vi "生成报表.vi"() -> ()   [LabVIEW 2013]
panel:
  in  "error in (no error) 2":errorcluster={"status"=TRUE, "code"=51111, "source"="路径不存在"}
  in  "error in (no error)":errorcluster={"status"=TRUE, "code"=51111, "source"="路径不存在"}
  out "String":string
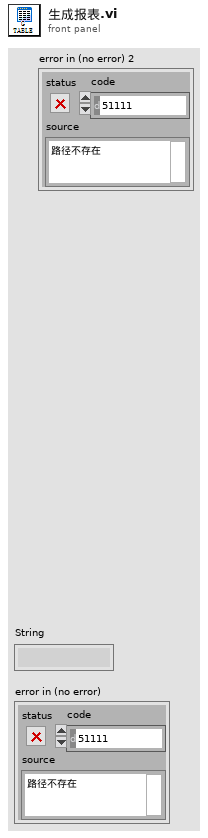
[diagram p1: front panel]
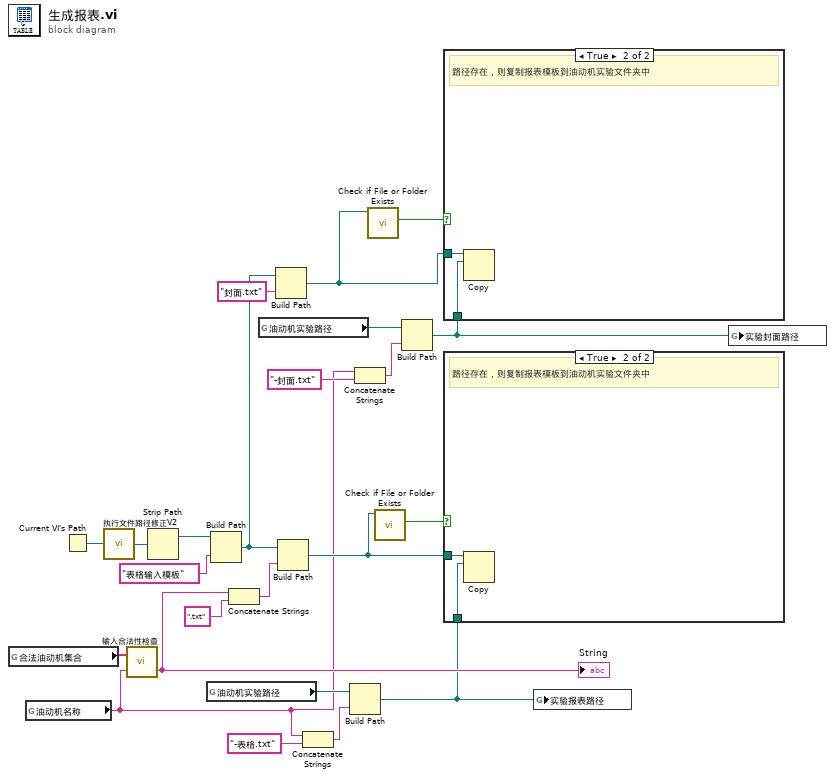
[diagram p0: block diagram]
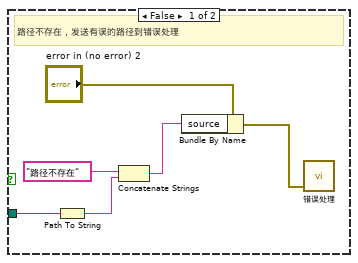
[diagram p2: hidden frame]
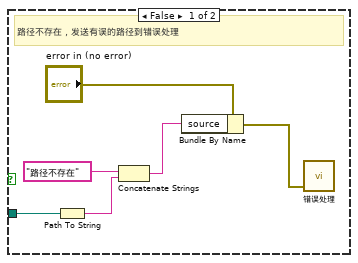
[diagram p3: hidden frame]
diagram:
  n1 = global read "合法油动机集合.vi" "合法油动机集合"() -> (w23:string[])
  n2 = global read "油动机名称.vi" "油动机名称"() -> (w2:string)
  n3 = Current VI's Path() -> (path=w11:path)
  n4 = call "执行文件路径修正V2.vi"("Path in"=w11) -> ("Path out"=w10:path)
  n5 = call "输入合法性检查.vi"("被检查名称"=w2, "合法名称集合"=w23) -> ("合法名称"=w15:string)  [unwired: 1 out]
  "String" <- w15
  n6 = Strip Path(path=w10) -> (stripped path=w22:path)  [unwired: 1 out]
  n7 = global read "油动机实验路径.vi" "油动机实验路径"() -> (w16:path)
  n8 = Build Path(base path=w22, name or relative path="表格输入模板" ("名称或相对路径")) -> (appended path=w8:path)
  n9 = Concatenate Strings(w15, ".txt" ("字符串")) -> (w19:string)
  n10 = global read "油动机实验路径.vi" "油动机实验路径"() -> (w3:path)
  n11 = Build Path(base path=w8, name or relative path="封面.txt") -> (appended path=w6:path)
  n12 = Build Path(base path=w8, name or relative path=w19) -> (appended path=w12:path)
  n13 = Concatenate Strings(w2, "-表格.txt" ("字符串")) -> (w17:string)
  n14 = Build Path(base path=w16, name or relative path=w17) -> (appended path=w14:path)
  n15 = Concatenate Strings(w2, "-封面.txt" ("字符串")) -> (w4:string)
  n16 = call <vilib>:"Check if File or Folder Exists.vi"("path"=w6) -> ("file or folder exists?"=w9:bool)  [unwired: 8 in, 2 out]
  n17 = call <vilib>:"Check if File or Folder Exists.vi"("path"=w12) -> ("file or folder exists?"=w13:bool)  [unwired: 8 in, 2 out]
  n18 = Build Path(base path=w3, name or relative path=w4) -> (appended path=w1:path)
  n19 = case shown="True" w9 {
    tunnel: w6 -> [w28 w31]
    tunnel: w1 -> [_ w30]
    frame False {
      # "路径不存在，发送有误的路径到错误处理"
      n20 = Path To String(path=w28) -> (string=w26:string)
      n21 = Concatenate Strings("路径不存在", w26) -> (w25:string)
      n22 = Bundle By Name(cluster="error in (no error) 2", "source"=w25) -> (w24:errorcluster)
      n23 = call "错误处理.vi"("error in (no error)"=w24) -> ()  [unwired: 2 in]
    }
    frame True {
      # "路径存在，则复制报表模板到油动机实验文件夹中"
      n24 = Copy(10:w30, 11:w31) -> ()  [unwired: 3 in, 3 out]
    }
  }
  n25 = case shown="True" w13 {
    tunnel: w12 -> [w36 w39]
    tunnel: w14 -> [_ w38]
    frame False {
      # "路径不存在，发送有误的路径到错误处理"
      n26 = Path To String(path=w36) -> (string=w34:string)
      n27 = Concatenate Strings("路径不存在", w34) -> (w33:string)
      n28 = Bundle By Name(cluster="error in (no error)", "source"=w33) -> (w32:errorcluster)
      n29 = call "错误处理.vi"("error in (no error)"=w32) -> ()  [unwired: 2 in]
    }
    frame True {
      # "路径存在，则复制报表模板到油动机实验文件夹中"
      n30 = Copy(10:w38, 11:w39) -> ()  [unwired: 3 in, 3 out]
    }
  }
  n31 = global write "实验报表路径.vi" "实验报表路径"(w14) -> ()
  n32 = global write "实验封面路径.vi" "实验封面路径"(w1) -> ()
